vi "B Spoof Relative Wind.vi"(6 "Wind Speed":dbl, 7 "Wind Angle":T1 format="%05.1f", 8 "Velocity (3 array)":dbl[](array[numeric])) -> (0 "Apparent Wind\nSpeed":T2, 1 "Perceived Wind":cluster{"X Position":dbl, "Y Position":dbl}, 2 "Apparent Wind\nDirection":T3, 3 "Global Wind":cluster{"X Position":dbl, "Y Position":dbl}, 5 "Robot\nHeading":T1 format="%05.1f")   [LabVIEW 2011]
uses:
  2-Think/2 Typedefs/heading.ctl
  2-Think/2 Typedefs/apparent wind direction.ctl
  2-Think/2 Typedefs/apparent wind speed.ctl
  <vilib>/Analysis/_algsub.llb/Real Vector Norm.vi
  <vilib>/Analysis/baseanly.llb/Real Dot Product.vi
  <vilib>/Analysis/NI_AALPro.lvlib
  <vilib>/Analysis/NI_AALBase.lvlib
panel:
  out "Heading Out":T1 format="%05.1f"
  out "Heading unit\nvector":cluster{"X Position":dbl, "Y Position":dbl}
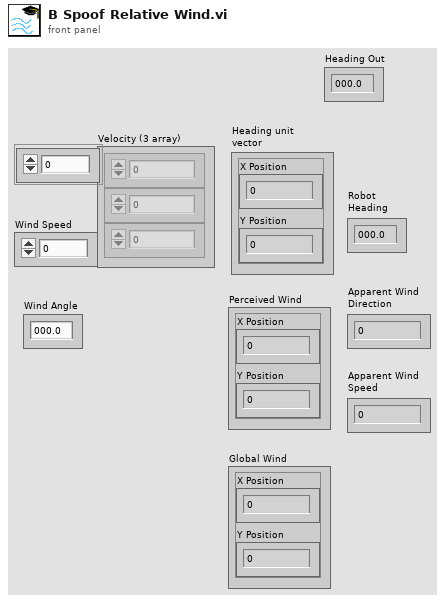
[diagram p1: front panel]
types:
  T1 = typedef "heading.ctl" = dbl
  T2 = typedef "apparent wind speed.ctl" = dbl
  T3 = typedef "apparent wind direction.ctl" = dbl
  T4 = typedef "Velocity.ctl" = cluster{"East":dbl, "North":dbl}
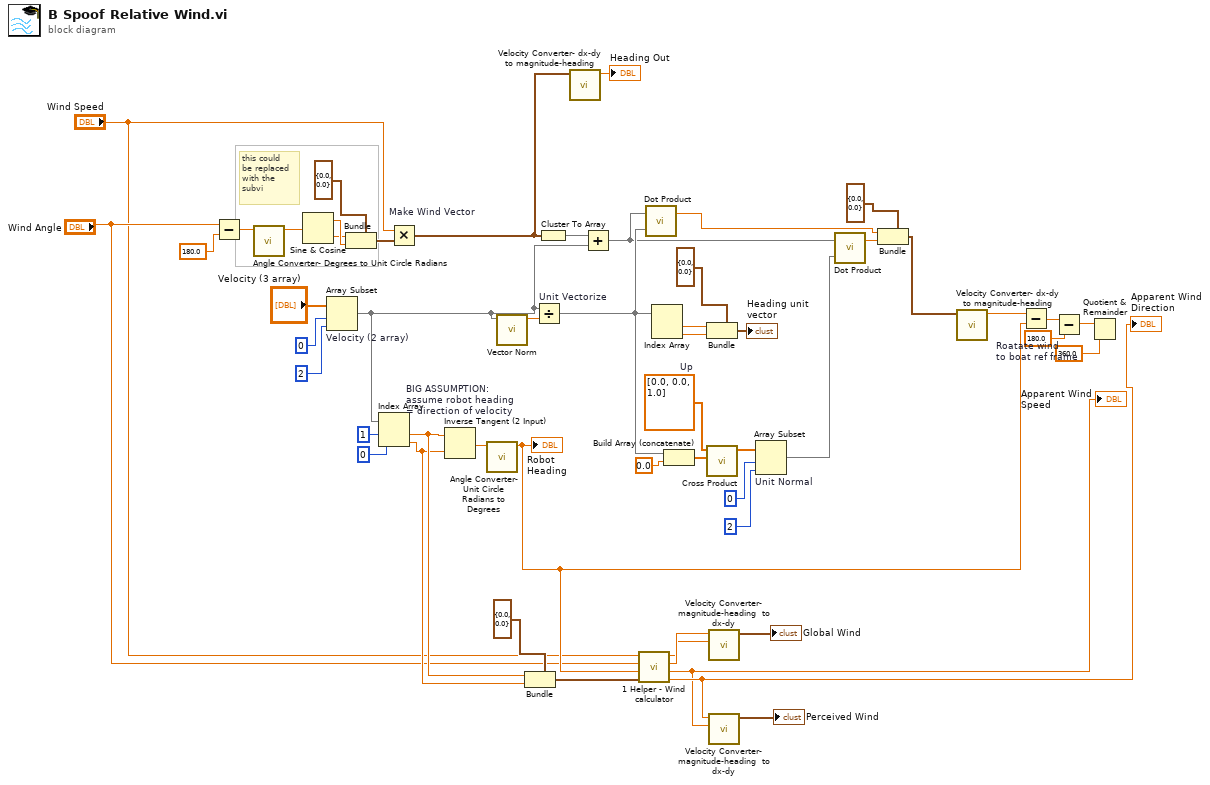
[diagram p0: block diagram]
diagram:
  w29 = dbl[] [0.0, 0.0, 1.0]  # Up
  # "this could\nbe replaced\nwith the\nsubvi"
  n1 = Subtract(x="Wind Angle", y=T1 180.0 ("Wind Angle 2")) -> (x-y=w27:T1)
  n2 = call "Angle Converter- Degrees to Unit Circle Radians.vi"("Angle in \nHeading \nFormat"=w27) -> ("Angle in \nUnit Circle\nRadians"=w28:dbl)  [unwired: 10 in]
  n3 = Sine & Cosine(0:w28) -> (1:w43:dbl, 2:w42:dbl)
  n4 = Array Subset "Velocity (2 array)"(array="Velocity (3 array)", index=0, length=2) -> (w24:dbl[])
  n5 = Bundle(cluster=cluster{"X Position":dbl, "Y Position":dbl} {"X Position"=0.0, "Y Position"=0.0} ("Robot Location"), "X Position"=w42, "Y Position"=w43) -> (w44:cluster{"X Position":dbl, "Y Position":dbl})
  n6 = Index Array(array=w24, index #1=1 ("index"), index #2=0 ("index")) -> (element #1=w11:dbl, element #2=w10:dbl)
  n7 = Multiply "Make Wind Vector"(x="Wind Speed", y=w44) -> (x*y=w15:cluster{"X Position":dbl, "Y Position":dbl})
  n8 = Inverse Tangent (2 Input) "BIG ASSUMPTION:\nassume robot heading\n= direction of velocity"(1:w10, 2:w11) -> (0:w25:dbl)
  n9 = call "Angle Converter- Unit Circle Radians to Degrees.vi"("Angle in \nUnit Circle\nRadians"=w25) -> ("Angle in \nHeading \nFormat"=w9:T1)  [unwired: 10 in]
  "Robot\nHeading" <- w9
  n10 = call-poly <vilib>:"Vector Norm.vi"("Input Vector"=w24) -> ("norm"=w53:dbl)  [unwired: 9 in, 1 out]
  n11 = Bundle(cluster=cluster{"X Position":dbl, "Y Position":dbl} {"X Position"=0.0, "Y Position"=0.0} ("Robot Location"), "X Position"=w11, "Y Position"=w10) -> (w12:cluster{"X Position":dbl, "Y Position":dbl})
  n12 = Divide "Unit Vectorize"(x=w24, y=w53) -> (x/y=w38:dbl[])
  n13 = Cluster To Array(cluster=w15) -> (array=w50:dbl[])
  n14 = call "Velocity Converter- dx-dy to magnitude-heading.vi"("Vector In"=w15) -> ("Heading Out"=→"Heading Out":T1)  [unwired: 9 in, 1 out]
  n15 = Add(x=w50, y=w24) -> (x+y=w33:dbl[])
  n16 = call "1 Helper - Wind calculator.vi"("Robot Velocity"=w12, "Heading"=w9, "Absolute Wind Direction"="Wind Angle", "Absolute Wind Speed"="Wind Speed") -> ("Apparent Wind Direction"=w6:T1, "Apparent Wind Speed"=w5:T2, "Absolute Wind Direction"=w3:T1, "Absolute Wind Speed"=w2:dbl)  [unwired: 4 in]
  "Apparent Wind\nDirection" <- w6
  "Apparent Wind\nSpeed" <- w5
  n17 = call-poly <vilib>:"Dot Product.vi"("Y Vector"=w38, "X Vector"=w33) -> ("X * Y"=w52:dbl)  [unwired: 1 out]
  n18 = Index Array(array=w38) -> (element #1=w47:dbl, element #2=w48:dbl)  [unwired: 2 in]
  n19 = Build Array (concatenate)(w38, 0.0) -> (w30:dbl[])
  n20 = Bundle(cluster=cluster{"X Position":dbl, "Y Position":dbl} {"X Position"=0.0, "Y Position"=0.0} ("Robot Location"), "X Position"=w47, "Y Position"=w48) -> (→"Heading unit\nvector":cluster{"X Position":dbl, "Y Position":dbl})
  n21 = call <vilib>:"Cross Product.vi"("B Vector"=w30, "A Vector"=w29) -> ("Cross Product"=w34:dbl[])  [unwired: 8 in, 1 out]
  n22 = call "Velocity Converter- magnitude-heading  to dx-dy.vi"("Magnitude"=w2, "Heading"=w3) -> ("Vector Out"=→"Global Wind":T4)  [unwired: 9 in]
  n23 = call "Velocity Converter- magnitude-heading  to dx-dy.vi"("Magnitude"=w5, "Heading"=w6) -> ("Vector Out"=→"Perceived Wind":T4)  [unwired: 9 in]
  n24 = Array Subset "Unit Normal"(array=w34, index=0, length=2) -> (w32:dbl[])
  n25 = call-poly <vilib>:"Dot Product.vi"("Y Vector"=w32, "X Vector"=w33) -> ("X * Y"=w31:dbl)  [unwired: 1 out]
  n26 = Bundle(cluster=cluster{"X Position":dbl, "Y Position":dbl} {"X Position"=0.0, "Y Position"=0.0} ("Perceived Wind"), "X Position"=w52, "Y Position"=w31) -> (w19:cluster{"X Position":dbl, "Y Position":dbl})
  n27 = call "Velocity Converter- dx-dy to magnitude-heading.vi"("Vector In"=w19) -> ("Heading Out"=w18:T1)  [unwired: 9 in, 1 out]
  n28 = Subtract "Roatate wind\nto boat ref frame"(x=w18, y=w9) -> (x-y=w21:T1)
  n29 = Subtract(x=w21, y=T1 180.0) -> (x-y=w17:T1)
  n30 = Quotient & Remainder(x=w17, y=T1 360.0) -> ()  [unwired: 2 out]
